vi "setProbeAttenuation.vi"(7 "Chn":string, 8 "error in (no error)":errorcluster, 10 "Attenuation":dbl=1.0, 11 "ScopeNi in":refnum<class "ScopeNi.lvclass">) -> (0 "error out":errorcluster, 3 "ScopeNi out":refnum<class "ScopeNi.lvclass">)   [LabVIEW 2023, in "ScopeNi.lvclass"]
doc: "<b>Author:</b> Wolfgang\n<b>Description:</b> configure the probe attenuation"
uses:
  ScopeNi.lvclass
  ScopeNi.lvclass/ScopeNi.ctl
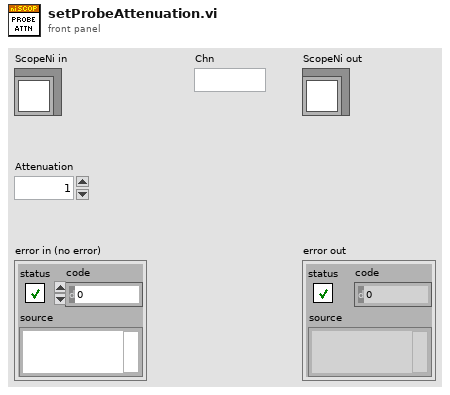
[diagram p1: front panel]
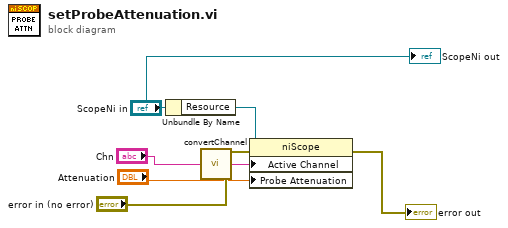
[diagram p0: block diagram]
diagram:
  n1 = Unbundle By Name("ScopeNi in") -> ("Resource"=w7:refnum<k15>)
  n2 = call "convertChannel.vi"("Chn in"="Chn") -> ("Chn out"=w1:string)
  n3 = property class="niScope"(reference=w7, error in="error in (no error)", "Active Channel"=w1, "Probe Attenuation"="Attenuation") -> (error out=→"error out":errorcluster)  [unwired: 1 out]
  "ScopeNi out" <- "ScopeNi in"
